vi "Status Bar.vi"(7 "action":T2=enum."Initialize", 8 "error in":errorcluster, 10 "Parameters":variant[](array[variant]), 11 "Devices":T1) -> (0 "error out":errorcluster, 3 "Status Bar":string)   [LabVIEW 2011]
uses:
  Status Bar.ctl
  Controls/Devices.ctl
  Modules/Hardware/Mass Flow Controller/Valve Status.ctl
  Modules/Hardware/Mass Flow Controller/Mass Flow Controller.lvclass
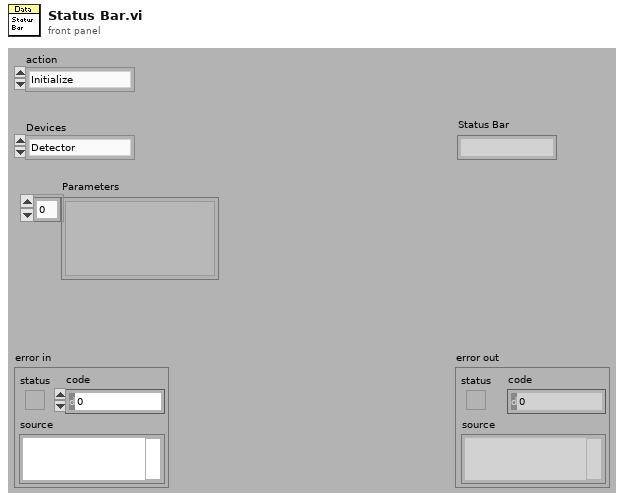
[diagram p1: front panel]
types:
  T1 = typedef "Devices.ctl" = enum16{"Detector", "Mass Flow Controller", "Power Supply"}
  T2 = typedef "Status Bar.ctl" = enum16{"Insert Into Status Bar", "Get Status Bar", "Initialize"}
  T3 = typedef "Mass Flow Controller.lvclass/Valve Status.ctl" = enum16{"Open", "Closed"}
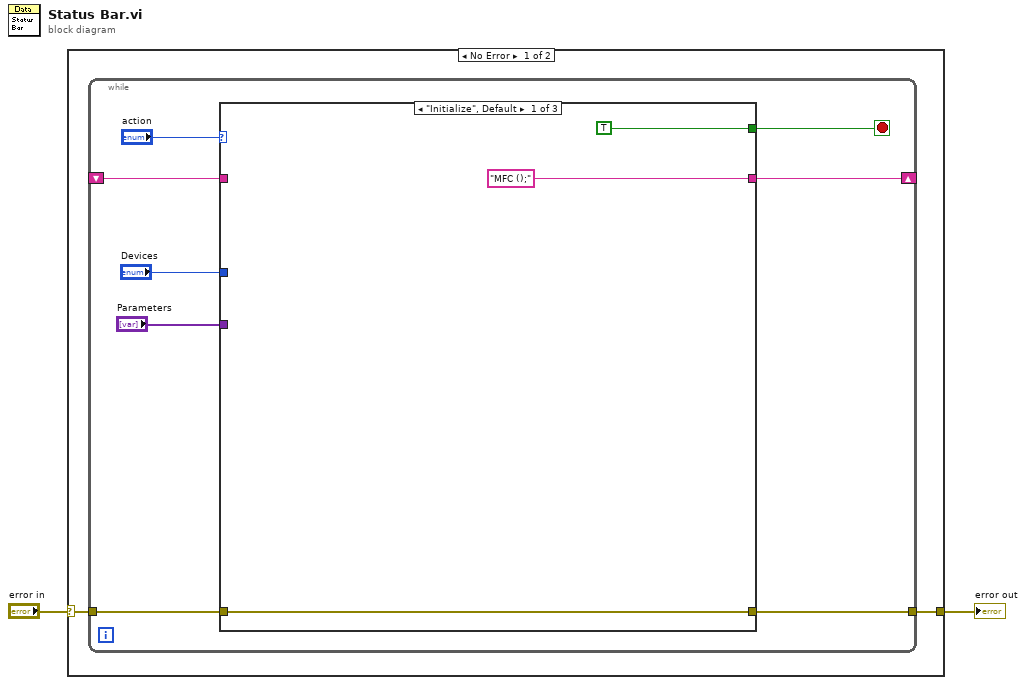
[diagram p0: block diagram]
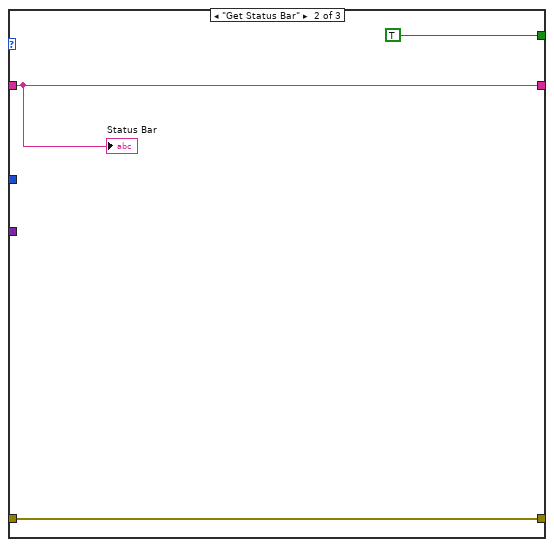
[diagram p2: hidden frame]
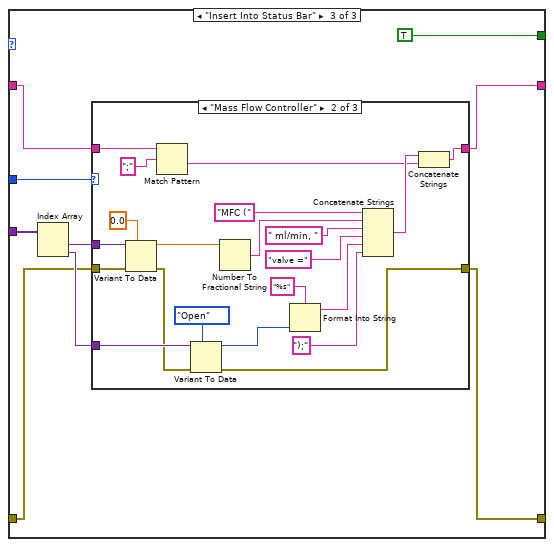
[diagram p3: hidden frame]
diagram:
  n1 = case shown="No Error" "error in" {
    selector: "error in" -> [w4 w53]
    tunnel: [w3 w53] -> w1
    frame No Error {
      n2 = while {
        tunnel: w4 -> [w11]
        tunnel: [w10] -> w3
        shift-right: [w8] -> _
        shift-left: _ -> [w7]
        stop <- w9 stop-if-true
        n3 = case shown="\"Initialize\", Default" "action" {
          tunnel: w11 -> [w15 w18 w22]
          tunnel: [w15 w18 w19] -> w10
          tunnel: [TRUE TRUE TRUE] -> w9
          tunnel: ["MFC ();" w16 w20] -> w8
          tunnel: w7 -> [_ w16 w21]
          tunnel: "Devices" -> [_ _ w26]
          tunnel: "Parameters" -> [_ _ w25]
          frame "Initialize", Default {
          }
          frame "Get Status Bar" {
            "Status Bar" <- w16
          }
          frame "Insert Into Status Bar" {
            n4 = Index Array(array=w25) -> (element #1=w24:variant, element #2=w23:variant)  [unwired: 2 in]
            n5 = case shown="\"Mass Flow Controller\"" w26 {
              tunnel: w24 -> [_ w50 _]
              tunnel: w23 -> [_ w48 _]
              tunnel: w22 -> [w28 w47 w52]
              tunnel: w21 -> [w29 w44 w51]
              tunnel: [w29 w31 w51] -> w20
              tunnel: [w28 w30 w52] -> w19
              frame "Detector", Default {
              }
              frame "Mass Flow Controller" {
                n6 = Variant To Data(error in=w47, type=0.0, Variant=w50) -> (data=w42:dbl, error out=w46:errorcluster)
                n7 = Match Pattern(string=w44, regular expression=";") -> (after substring=w32:string)  [unwired: 1 in, 3 out]
                n8 = Variant To Data(error in=w46, type=Valve_Status."Open" ("Valve Status"), Variant=w48) -> (data=w37:T3, error out=w30:errorcluster)
                n9 = Number To Fractional String(number=w42) -> (F-format string=w40:string)  [unwired: 3 in]
                n10 = Format Into String(format string="%s", w37) -> (resulting string=w35:string)  [unwired: 2 in, 1 out]
                n11 = Concatenate Strings("MFC (" ("string"), w40, " ml/min, " ("string"), "valve =" ("string"), w35, ");" ("string")) -> (w33:string)
                n12 = Concatenate Strings(w33, w32) -> (w31:string)
              }
              frame "Power Supply" {
              }
            }
          }
        }
      }
    }
    frame Error {
    }
  }
  "error out" <- w1
